vi "Radial Calculation.vi"(0 "Power":dbl, 1 "X":dbl[](array[numeric]), 11 "Thikness":dbl, 12 "Y":dbl[](array[numeric])) -> (3 "K4-5":dbl, 4 "K2-3":dbl, 6 "K1-2":dbl, 10 "XY Graph":cluster{"Ramp Pattern":dbl[], dbl[]}[](graph), 14 "K3-4":dbl, 15 "Result":dbl)   [LabVIEW 2017]
uses:
  <vilib>/express/express arith-compare/Formula/XNode/ExpressFormulaBlockNode.xnode
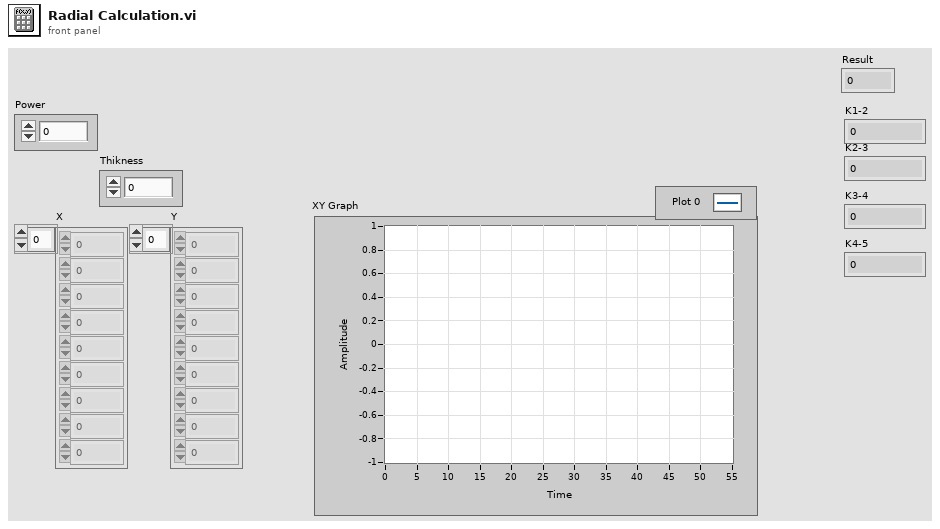
[diagram p1: front panel]
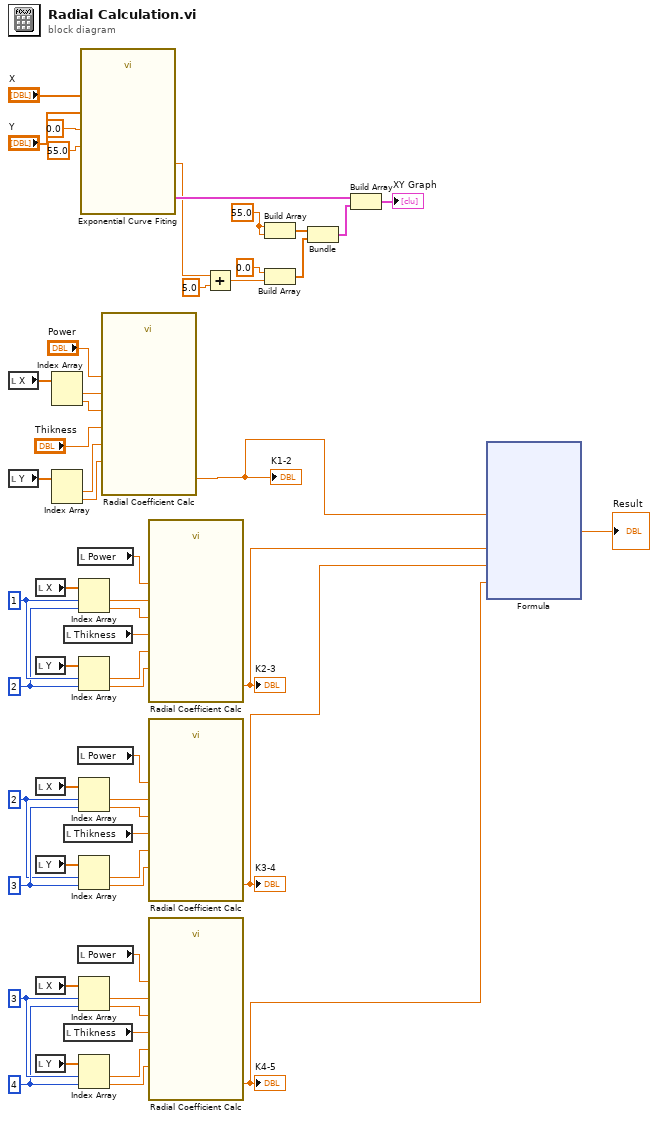
[diagram p0: block diagram]
diagram:
  w8 = 4 ("index")
  w9 = 3 ("index")
  w25 = 3 ("index")
  w24 = 2 ("index")
  w28 = 2 ("index")
  w29 = 1 ("index")
  w52 = 55.0 ("element")
  n1 = local read "X"() -> (w42:dbl[])
  n2 = local read "Y"() -> (w39:dbl[])
  n3 = local read "X"() -> (w31:dbl[])
  n4 = local read "Y"() -> (w34:dbl[])
  n5 = local read "X"() -> (w22:dbl[])
  n6 = local read "Y"() -> (w19:dbl[])
  n7 = local read "X"() -> (w11:dbl[])
  n8 = local read "Y"() -> (w14:dbl[])
  n9 = Index Array(array=w42) -> (element #1=w41:dbl, element #2=w40:dbl)  [unwired: 2 in]
  n10 = Index Array(array=w39) -> (element #1=w38:dbl, element #2=w37:dbl)  [unwired: 2 in]
  n11 = local read "Thikness"() -> (w27:dbl)
  n12 = local read "Thikness"() -> (w26:dbl)
  n13 = local read "Thikness"() -> (w7:dbl)
  n14 = local read "Power"() -> (w30:dbl)
  n15 = local read "Power"() -> (w23:dbl)
  n16 = local read "Power"() -> (w10:dbl)
  n17 = Index Array(array=w31, index #1=w29, index #2=w28) -> (element #1=w32:dbl, element #2=w33:dbl)
  n18 = Index Array(array=w34, index #1=w29, index #2=w28) -> (element #1=w35:dbl, element #2=w36:dbl)
  n19 = Index Array(array=w22, index #1=w24, index #2=w25) -> (element #1=w21:dbl, element #2=w20:dbl)
  n20 = Index Array(array=w19, index #1=w24, index #2=w25) -> (element #1=w18:dbl, element #2=w17:dbl)
  n21 = Index Array(array=w11, index #1=w9, index #2=w8) -> (element #1=w12:dbl, element #2=w13:dbl)
  n22 = Index Array(array=w14, index #1=w9, index #2=w8) -> (element #1=w15:dbl, element #2=w16:dbl)
  n23 = call "Exponential Curve Fiting.vi"("end"=55.0, "start"=0.0, "Y"="Y", "X"="X") -> ("T First"=w6:dbl, "XY Graph"=w46:cluster{"Ramp Pattern":dbl[], dbl[]})  [unwired: 1 in, 1 out]
  n24 = call "Radial Coefficient Calc.vi"("T2"=w37, "T1"=w38, "Power"="Power", "Thikness"="Thikness", "ri"=w41, "ro"=w40) -> ("K"=w5:dbl)
  "K1-2" <- w5
  n25 = call "Radial Coefficient Calc.vi"("T2"=w36, "T1"=w35, "Power"=w30, "Thikness"=w27, "ri"=w32, "ro"=w33) -> ("K"=w4:dbl)
  "K2-3" <- w4
  n26 = call "Radial Coefficient Calc.vi"("T2"=w17, "T1"=w18, "Power"=w23, "Thikness"=w26, "ri"=w21, "ro"=w20) -> ("K"=w3:dbl)
  "K3-4" <- w3
  n27 = call "Radial Coefficient Calc.vi"("T2"=w16, "T1"=w15, "Power"=w10, "Thikness"=w7, "ri"=w12, "ro"=w13) -> ("K"=w2:dbl)
  "K4-5" <- w2
  n28 = Add(x=w6, y=5.0) -> (x+y=w50:dbl)
  n29 = Build Array(w52, w52) -> (w48:dbl[])
  n30 = Build Array(0.0 ("element"), w50) -> (w47:dbl[])
  n31 = Bundle(w48, w47) -> (w45:cluster{dbl[], dbl[]})  [unwired: 1 in]
  n32 = Build Array(w46, w45) -> (→"XY Graph":cluster{"Ramp Pattern":dbl[], dbl[]}[])
  n33 = xnode "Formula"("X1"=w5, "X2"=w4, "X3"=w3, "X4"=w2) -> ("Result"=→"Result":dbl)  [unwired: 1 in, 1 out]
